vi "Get Angle.vi"(6 "Axis":T1, 8 "error in (no error)":errorcluster, 11 "Instrument.Cryostat in":refnum<class "Instrument.Cryostat.lvclass">) -> (0 "error out":errorcluster, 1 "Status":string, 2 "Angle (°)":dbl, 3 "Instrument.Cryostat out":refnum<class "Instrument.Cryostat.lvclass">)   [LabVIEW 2019, in "Instrument.Cryostat.lvclass"]
uses:
  Instrument.Cryostat.lvclass
  Typedefs/Rotator Axis--Enum.ctl
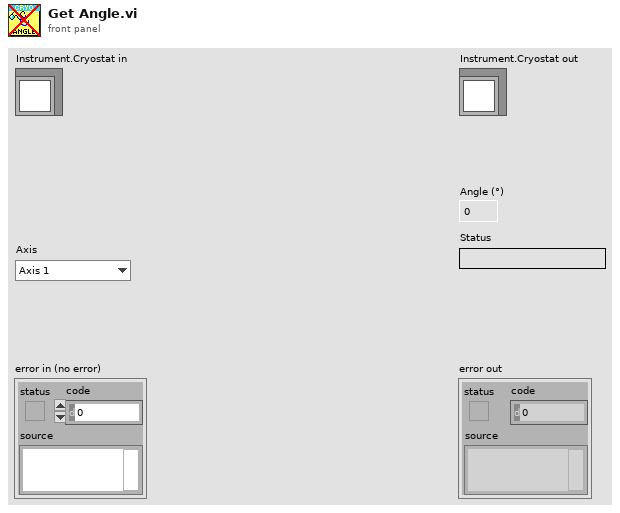
[diagram p1: front panel]
types:
  T1 = typedef "Instrument.Cryostat.lvclass/Rotator Axis--Enum.ctl" = enum16{"Axis 1", "Axis 2"}
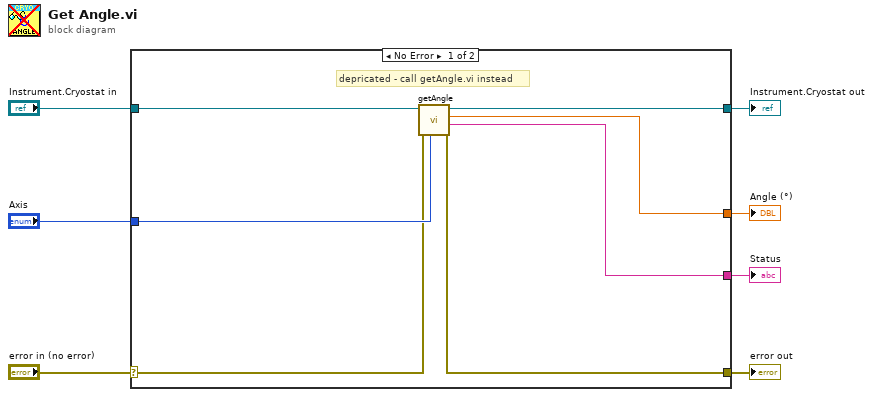
[diagram p0: block diagram]
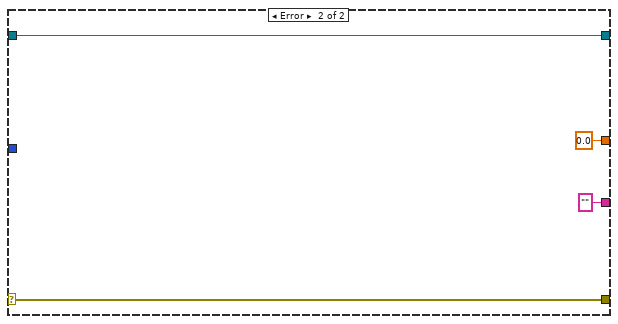
[diagram p2: hidden frame]
diagram:
  n1 = case shown="No Error" "error in (no error)" {
    selector: "error in (no error)" -> [w11 w18]
    tunnel: [w10 w18] -> w6
    tunnel: [w14 w17] -> w4
    tunnel: "Instrument.Cryostat in" -> [w13 w17]
    tunnel: "Axis" -> [w12 _]
    tunnel: [w9 0.0 ("Angle (°)")] -> w2
    tunnel: [w8 "" ("Status")] -> w1
    frame No Error {
      # "depricated - call getAngle.vi instead"
      n2 = call-dynamic "getAngle.vi"("Channel"=w12, "error in (no error)"=w11, "Instrument.Cryostat in"=w13) -> ("error out"=w10:errorcluster, "Status"=w8:string, "Angle (°)"=w9:dbl, "Instrument.Cryostat out"=w14:refnum<class "Instrument.Cryostat.lvclass">)  [unwired: 5 in]
    }
    frame Error {
    }
  }
  "error out" <- w6
  "Instrument.Cryostat out" <- w4
  "Angle (°)" <- w2
  "Status" <- w1
